vi "Rollover Events.vi"() -> ()   [LabVIEW 2018]
uses:
  src/api/logger_class/Log Levels.ctl
  bc269cd9-d162-4013-a312-bd866d79ee19.vi
  src/api/configuration/handlers/file_handler/File Handler.lvclass
  C:/Users/Colin/Documents/software_projects/labview/glog/src/api/extension/formatting_handler_interface/Formatting Handler.lvclass
  src/api/logger_class/Log (Parts).vi
  src/api/logger_class/Logger.lvclass
panel:
  in  "Stop":bool
  out "Source":string
  out "Current Log File":path
  out "sources":string[](array[string])
  out "log files":path[](array[path])
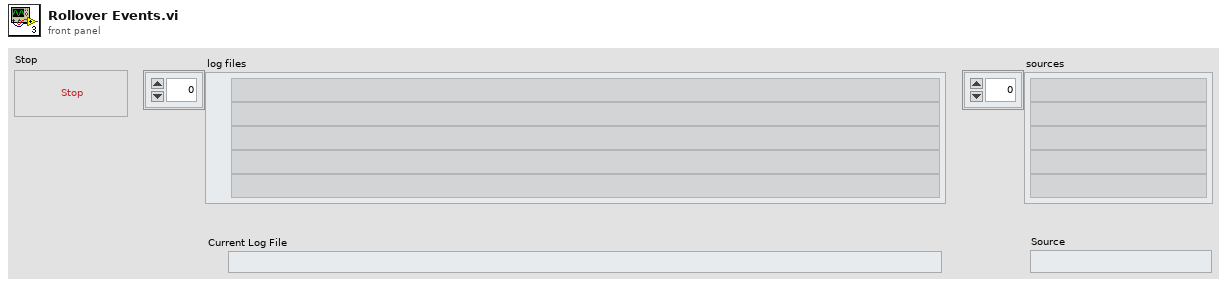
[diagram p1: front panel]
types:
  T1 = typedef "GLog.lvlib/File Handler.lvclass/Events.ctl" = cluster{"File Rollover":refnum<user-event>}
  T2 = typedef "GLog.lvlib/Logger.lvclass/Log Levels.ctl" = enum16{"Trace", "Debug", "Info", "Warning", "Error", "Critical"}
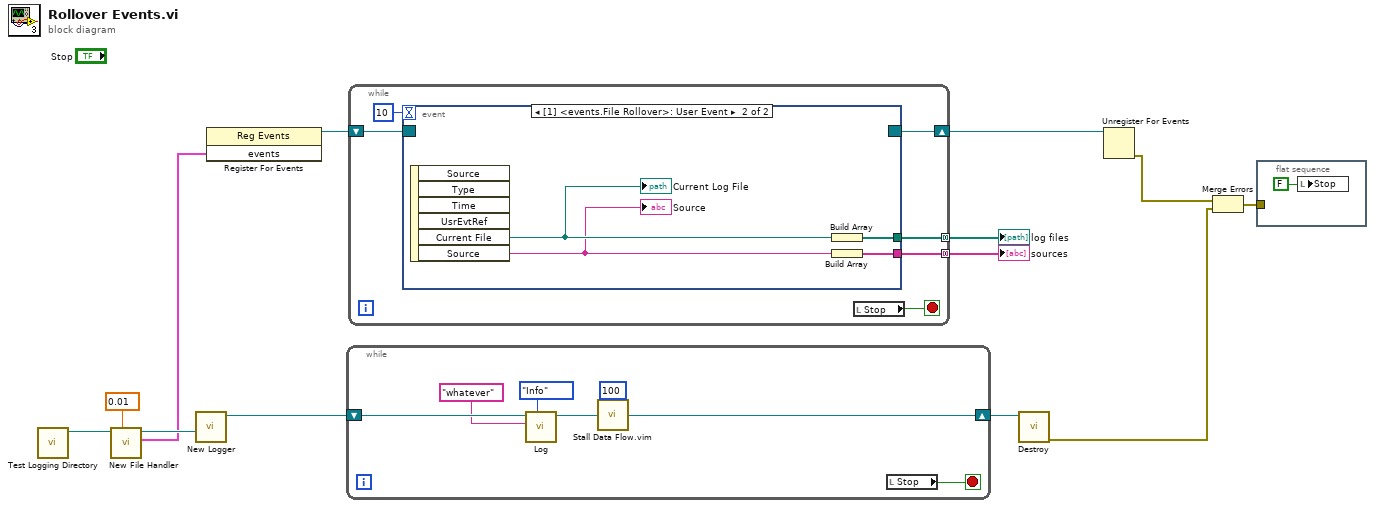
[diagram p0: block diagram]
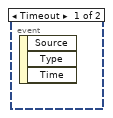
[diagram p2: hidden frame]
diagram:
  n1 = call "Test Logging Directory.vi"() -> ("test logging directory"=w11:path)  [unwired: 11 in]
  n2 = call "New File Handler.vi"("max file size [MB](50)"=0.01, "log directory (<app dir>/logs)"=w11) -> ("events"=w10:T1, "file handler"=w13:refnum<class "File Handler.lvclass">)  [unwired: 7 in, 1 out]
  n3 = call "New Logger.vi"("log handler (file handler)"=w13) -> ("logger"=w6:refnum<class "Logger.lvclass">)  [unwired: 9 in, 1 out]
  n4 = register-events(w10) -> (reference out=w9:refnum<event-registration>)  [unwired: 2 in, 1 out]
  n5 = while {
    shift-right: [w17] -> w5
    shift-left: w6 -> [w20]
    stop <- w15 stop-if-true
    n6 = call-poly "Log.vi"("log level"=Log_Levels."Info", "message"="whatever", "logger in"=w20) -> ("logger out"=w18:refnum<class "Logger.lvclass">)  [unwired: 8 in]
    n7 = call "Stall Data Flow.vim"("value in"=w18, "milliseconds to wait"=u32 100) -> ("value out"=w17:refnum<class "Logger.lvclass">)  [unwired: 1 out]
    n8 = local read "Stop"() -> (w15:bool)
  }
  n9 = while {
    shift-right: [w25] -> w4
    shift-left: w9 -> [w26]
    tunnel: [w24] -> w8 mode=concatenating
    tunnel: [w23] -> w7 mode=concatenating
    stop <- w22 stop-if-true
    n10 = event shown="[1] <events.File Rollover>: User Event" {
      selector: w26 -> [_ _]
      dyn-events: [_ _] -> w25
      timeout: 10 -> [_ _]
      tunnel: [_ w28] -> w24
      tunnel: [_ w27] -> w23
      event Timeout {
        n11 = event-data() -> ()  [unwired: 1 in, 3 out]
      }
      event User Event {
        n12 = event-data() -> ("Current File"=w30:path, "Source"=w29:string)  [unwired: 1 in, 4 out]
        "Current Log File" <- w30
        "Source" <- w29
        n13 = Build Array(w30) -> (w28:path[])
        n14 = Build Array(w29) -> (w27:string[])
      }
    }
    n15 = local read "Stop"() -> (w22:bool)
  }
  "log files" <- w8
  "sources" <- w7
  n16 = call "Destroy.vi"("logger in"=w5) -> ("error out"=w2:errorcluster)  [unwired: 9 in, 1 out]
  n17 = Unregister For Events(event registration refnum=w4) -> (error out=w3:errorcluster)  [unwired: 1 in]
  n18 = Merge Errors(w3, w2) -> (w1:errorcluster)
  n19 = flat-sequence {
    tunnel: w1 -> [_]
    frame #0 {
      n20 = local write "Stop"(FALSE ("Stop")) -> ()
    }
  }
